vi "getStrain.vi"(6 "Channel":i32, 8 "error in (no error)":errorcluster, 11 "Instrument.Strain in":refnum<class "Instrument.Strain.lvclass">) -> (0 "error out":errorcluster, 2 "Strain (V)":dbl, 3 "Instrument.Strain out":refnum<class "Instrument.Strain.lvclass">)   [LabVIEW 2019, in "Instrument.Strain.lvclass"]
uses:
  Instrument.Strain.lvclass
  Instrument/Instrument.lvclass
  2ed86b82-ed51-4baf-a53c-8bd0a09ce437.vi
  C:/Users/patrick/Documents/GitHub/Instrument-Framework/lvsrc/Instrument/Instrument.lvclass
  C:/Program Files (x86)/National Instruments/LabVIEW 2019/vi.lib/JKI/JKI SMO/SMO/SMO.lvclass
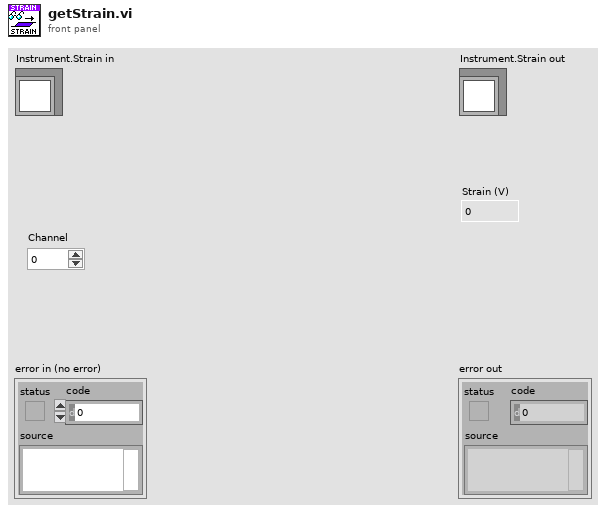
[diagram p1: front panel]
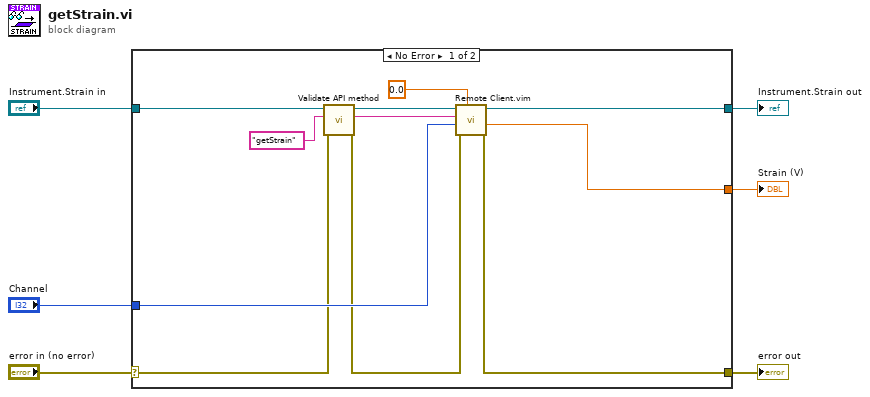
[diagram p0: block diagram]
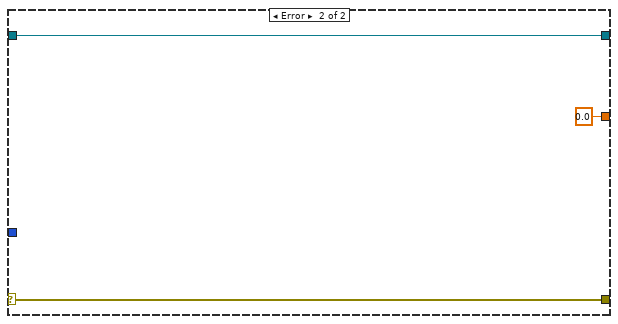
[diagram p2: hidden frame]
diagram:
  n1 = case shown="No Error" "error in (no error)" {
    selector: "error in (no error)" -> [w12 w20]
    tunnel: [w11 w20] -> w5
    tunnel: [w13 w19] -> w3
    tunnel: "Instrument.Strain in" -> [w15 w19]
    tunnel: "Channel" -> [w14 _]
    tunnel: [w8 0.0 ("Data out")] -> w1
    frame No Error {
      n2 = call "Validate API method.vi"("error in (no error)"=w12, "Command in"="getStrain" ("error message (\"\")"), "Instrument in"=w15) -> ("error out"=w10:errorcluster, "command out"=w7:string, "Instrument out"=w16:refnum<class "Instrument.Strain.lvclass">)  [unwired: 6 in]
      n3 = call "Remote Client.vim"("Command out"=w7, "Data Out type"=0.0, "error in (no error)"=w10, "Data in"=w14, "Instrument in"=w16) -> ("error out"=w11:errorcluster, "Data out"=w8:dbl, "Instrument out"=w13:refnum<class "Instrument.Strain.lvclass">)  [unwired: 4 in]
    }
    frame Error {
    }
  }
  "error out" <- w5
  "Instrument.Strain out" <- w3
  "Strain (V)" <- w1
